vi "Clear_DAQ_Tasks.vi"(8 "error in (no error)":errorcluster, 11 "Data Cluster":T1) -> (0 "error out":errorcluster)   [LabVIEW 2017]
uses:
  Controls/ShiftRegisterCluster.ctl
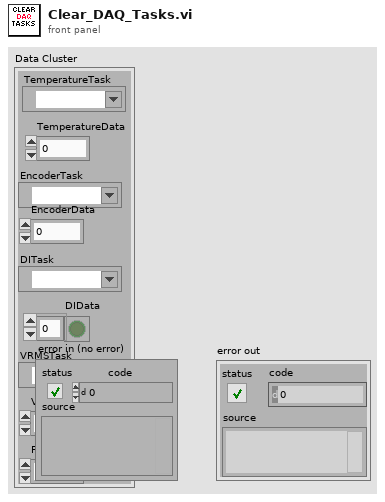
[diagram p1: front panel]
types:
  T1 = typedef "ShiftRegisterCluster.ctl" = cluster{"TemperatureTask":refnum<k21>, "TemperatureData":dbl, "EncoderTask":refnum<k21>, "EncoderData":dbl, "DITask":refnum<k21>, "DIData":bool[], "VRMSTask":refnum<k21>, "VRMSData":dbl, "FreqData":dbl}
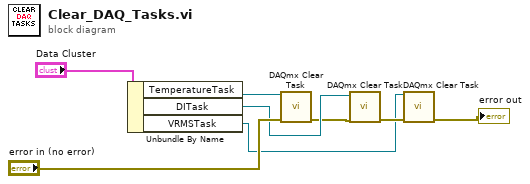
[diagram p0: block diagram]
diagram:
  n1 = Unbundle By Name("Data Cluster") -> ("TemperatureTask"=w8:refnum<k21>, "DITask"=w5:refnum<k21>, "VRMSTask"=w1:refnum<k21>)
  n2 = call <vilib>:"DAQmx Clear Task.vi"("task in"=w8, "error in"="error in (no error)") -> ("error out"=w4:errorcluster)  [unwired: 13 in]
  n3 = call <vilib>:"DAQmx Clear Task.vi"("task in"=w5, "error in"=w4) -> ("error out"=w3:errorcluster)  [unwired: 13 in]
  n4 = call <vilib>:"DAQmx Clear Task.vi"("task in"=w1, "error in"=w3) -> ("error out"=→"error out":errorcluster)  [unwired: 13 in]
